vi "GPS -Warn Audited Addr.vi"(0 "ctlMode4GPSTool":T1, 1 "LatPin":string, 2 "LngPin":string, 3 "AddrLat":dbl, 4 "AddrLng":dbl, 8 "Audited":bool) -> (12 "tbCtlGUI":enum32{"Position", "Pin Drop", "Addr", "Setup"}(ring), 14 "AddrLat -Out":dbl, 15 "AddrLng -OUT":dbl, 17 "LatPin":dbl, 18 "LngPin":dbl)   [LabVIEW 2019]
uses:
  ctlMode4GPSTool.ctl
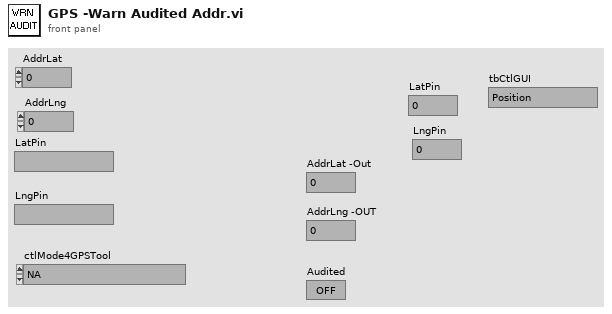
[diagram p1: front panel]
types:
  T1 = typedef "ctlMode4GPSTool.ctl" = enum16{"NA", "Audit"}
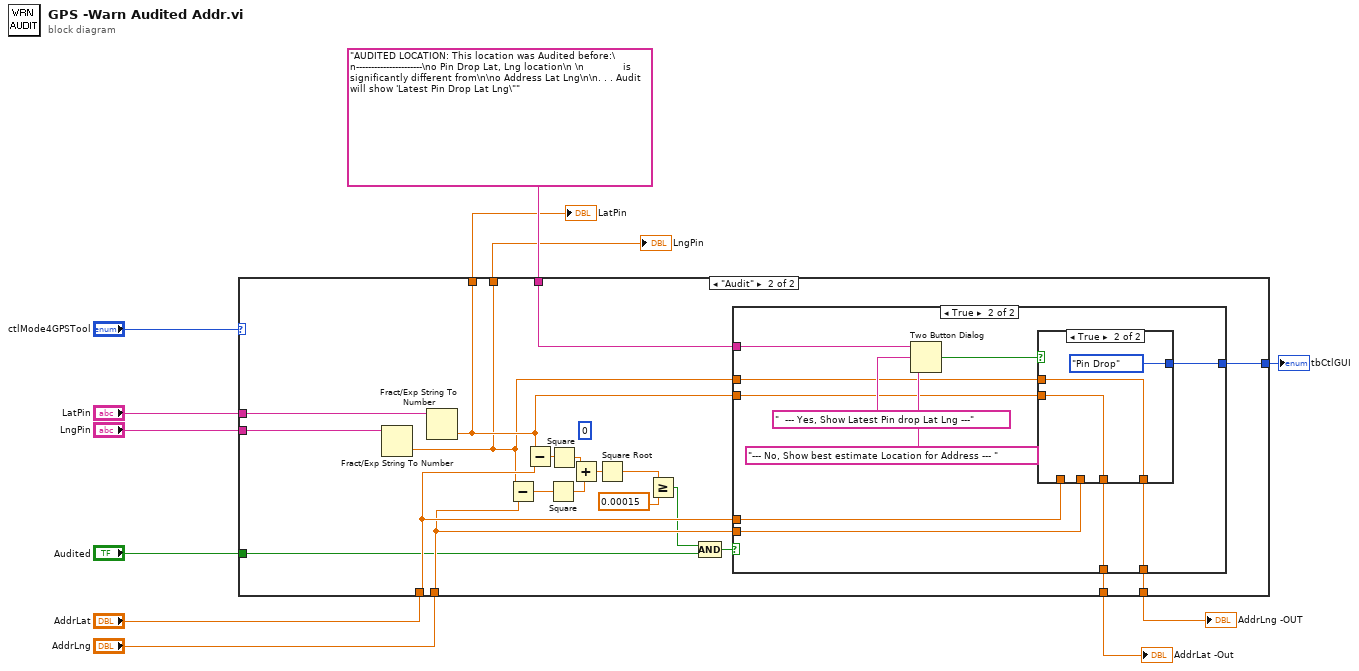
[diagram p0: block diagram]
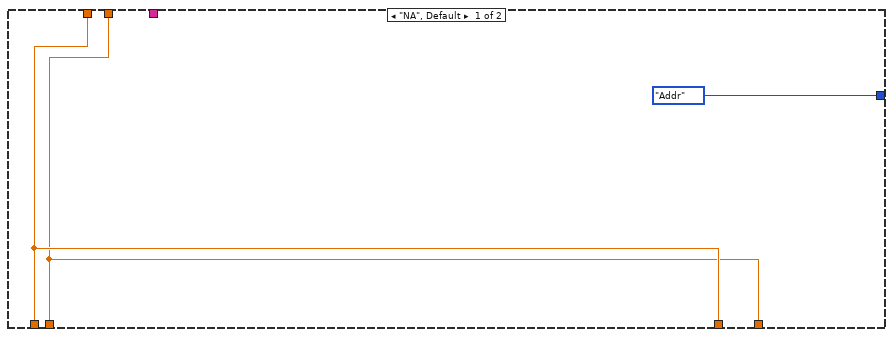
[diagram p2: hidden frame]
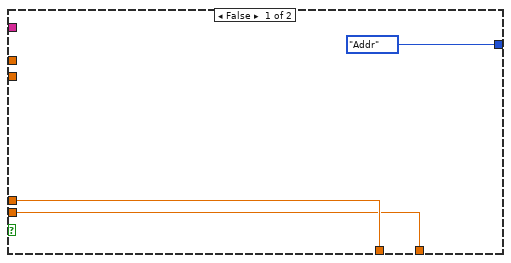
[diagram p3: hidden frame]
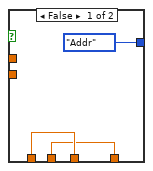
[diagram p4: hidden frame]
diagram:
  n1 = case shown="\"Audit\"" "ctlMode4GPSTool" {
    tunnel: "LatPin" -> [_ w20]
    tunnel: "LngPin" -> [_ w19]
    tunnel: "Audited" -> [_ w22]
    tunnel: "AddrLat" -> [w15 w27]
    tunnel: "AddrLng" -> [w14 w26]
    tunnel: "AUDITED LOCATION: This location was Audited before:\n----------------------\no Pin Drop Lat, Lng location\n \n             is significantly different from\n\no Address Lat Lng\n\n. . . Audit will show 'Latest Pin Drop Lat Lng\"" ("message") -> [_ w28]
    tunnel: [w15 w25] -> w4
    tunnel: [w14 w24] -> w5
    tunnel: [w15 w18] -> w3
    tunnel: [w14 w17] -> w2
    tunnel: [enum32{"Position", "Pin Drop", "Addr", "Setup"}."Addr" ("tbCtlGUI") w16] -> w1
    frame "NA", Default {
    }
    frame "Audit" {
      (unwired) 0
      n2 = Fract/Exp String To Number(string=w19) -> (number=w17:dbl)  [unwired: 3 in, 1 out]
      n3 = Fract/Exp String To Number(string=w20) -> (number=w18:dbl)  [unwired: 3 in, 1 out]
      n4 = Subtract(x=w17, y=w26) -> (x-y=w32:dbl)
      n5 = Subtract(x=w18, y=w27) -> (x-y=w31:dbl)
      n6 = Square(x=w32) -> (x^2=w33:dbl)
      n7 = Square(x=w31) -> (x^2=w34:dbl)
      n8 = Add(x=w34, y=w33) -> (x+y=w35:dbl)
      n9 = Square Root(x=w35) -> (sqrt(x)=w29:dbl)
      n10 = Greater Or Equal?(x=w29, y=0.00015) -> (x >= y?=w23:bool)
      n11 = Compound Arithmetic op=AND(w23, w22) -> (w21:bool)
      n12 = case shown="True" w21 {
        tunnel: w28 -> [_ w49]
        tunnel: w27 -> [w38 w41]
        tunnel: w26 -> [w37 w40]
        tunnel: w18 -> [_ w45]
        tunnel: w17 -> [_ w43]
        tunnel: [w38 w44] -> w25
        tunnel: [w37 w42] -> w24
        tunnel: [enum32{"Position", "Pin Drop", "Addr", "Setup"}."Addr" ("tbCtlGUI") w39] -> w16
        frame False {
        }
        frame True {
          n13 = Two Button Dialog(message=w49, 1:"--- No, Show best estimate Location for Address --- " ("T button name (\"OK\")"), 2:"  --- Yes, Show Latest Pin drop Lat Lng ---" ("T button name (\"OK\")")) -> (T button?=w46:bool)
          n14 = case shown="True" w46 {
            tunnel: w45 -> [_ w55]
            tunnel: [w52 w55] -> w44
            tunnel: [w51 w54] -> w42
            tunnel: w43 -> [_ w54]
            tunnel: w41 -> [w52 _]
            tunnel: w40 -> [w51 _]
            tunnel: [enum32{"Position", "Pin Drop", "Addr", "Setup"}."Addr" ("tbCtlGUI") enum32{"Position", "Pin Drop", "Addr", "Setup"}."Pin Drop" ("tbCtlGUI")] -> w39
            frame False {
            }
            frame True {
            }
          }
        }
      }
    }
  }
  "AddrLng -OUT" <- w5
  "AddrLat -Out" <- w4
  "LatPin" <- w3
  "LngPin" <- w2
  "tbCtlGUI" <- w1
